vi "Create MS Request Message Data .vi"(11 "MS Requested State":T1) -> (3 "MS State":string)   [LabVIEW 2016, in "TLMB.lvlib"]
uses:
  Projects/TLMB.lvlib
  type defs/Mode Shift Requested State.ctl
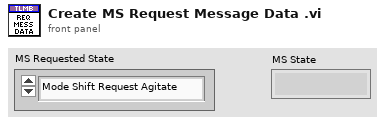
[diagram p1: front panel]
types:
  T1 = typedef "TLMB.lvlib/Mode Shift Requested State.ctl" = enum16{"Mode Shift Request Agitate", "Mode Shift Request Spin"}
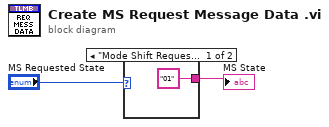
[diagram p0: block diagram]
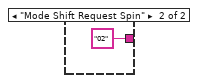
[diagram p2: hidden frame]
diagram:
  n1 = case shown="\"Mode Shift Request Agitate\", Default" "MS Requested State" {
    tunnel: ["01" "02"] -> w2
    frame "Mode Shift Request Agitate", Default {
    }
    frame "Mode Shift Request Spin" {
    }
  }
  "MS State" <- w2
